vi "obtain_trigger_queue.vi"(8 "error in (no error)":errorcluster, 11 "Stimulator090724Scaffold in":refnum<class "Stimulator090724Scaffold.lvclass">) -> (0 "error out":errorcluster, 2 "trigger queue":refnum<queue>, 3 "Stimulator090724Scaffold out":refnum<class "Stimulator090724Scaffold.lvclass">)   [LabVIEW 2010]
uses:
  StimulatorDL090724Scaffold.lvsc/Trigger.ctl
  StimulatorDL090724Scaffold.lvsc
  GenericStimulator/GenericStimulator/class_data.vi
  GenericStimulator/GenericStimulator/GenericStimulator.lvclass
  Stimulator090724Scaffold.lvclass
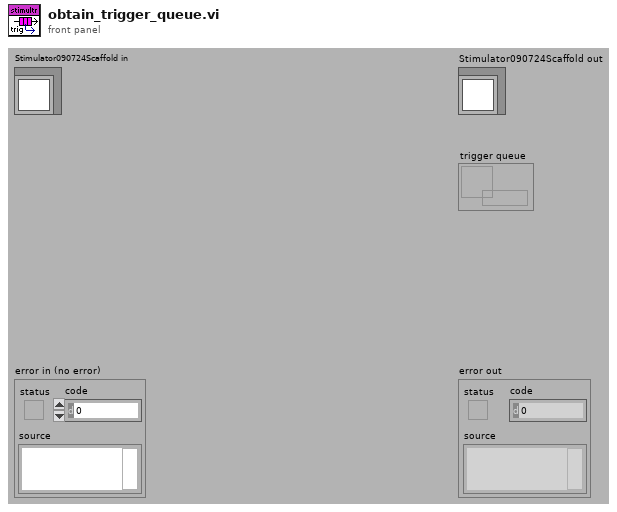
[diagram p1: front panel]
types:
  T1 = typedef "StimulatorDL090724Scaffold.lvsc/Trigger.ctl" = enum16{"NULL", "initialise", "terminate", "start sweep", "stop sweep", "start continuous stimulation", "stop continuous stimulation"}
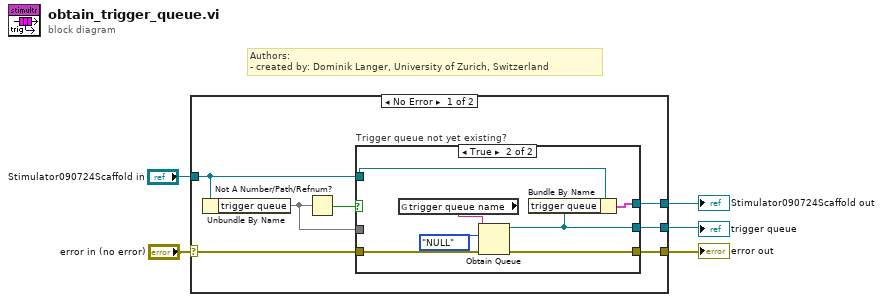
[diagram p0: block diagram]
diagram:
  # "Authors: \n- created by: Dominik Langer, University of Zurich, Switzerland"
  n1 = case shown="No Error" "error in (no error)" {
    selector: "error in (no error)" -> [w12 w24]
    tunnel: [w11 w24] -> w4
    tunnel: [w9 w23] -> w2
    tunnel: "Stimulator090724Scaffold in" -> [w8 w23]
    tunnel: [w10 _] -> w1
    frame No Error {
      n2 = Unbundle By Name(w8) -> ("trigger queue"=w6)
      n3 = Not A Number/Path/Refnum?(number/path/refnum=w6) -> (NaN/Path/Refnum?=w7:bool)
      n4 = case "Trigger queue not yet existing?" shown="True" w7 {
        tunnel: w12 -> [w13 w21]
        tunnel: [w13 w20] -> w11
        tunnel: [w15 w18] -> w10
        tunnel: w8 -> [w14 w17]
        tunnel: [w14 w16] -> w9
        tunnel: w6 -> [w15 _]
        frame False {
        }
        frame True {
          n5 = global read "class_data.vi" "trigger queue name"() -> (w19:string)
          n6 = Obtain Queue(name (unnamed)=w19, element data type=Trigger."NULL" ("Trigger"), error in (no error)=w21) -> (queue out=w18:refnum<queue>, error out=w20:errorcluster)  [unwired: 2 in, 1 out]
          n7 = Bundle By Name(cluster=w17, "trigger queue"=w18) -> (w16:cluster{})
        }
      }
    }
    frame Error {
    }
  }
  "error out" <- w4
  "Stimulator090724Scaffold out" <- w2
  "trigger queue" <- w1
